vi "IMAQ Trigger the captured image.vi"() -> ()   [LabVIEW 2018]
uses:
  LabViewDVPCamera/LabViewDVPCamera.lvlib
panel:
  out "Image":T1(plugin-control)
  in  "Trigger":bool
  in  "CloseFlg":i32
  out "handle":u32
  in  "CameraList":u16(ring) items=["MGS130M-192.168.0.251"]
  in  "Set":bool
  in  "Close":bool
  in  "Open":bool
  in  "ScanCamera":bool
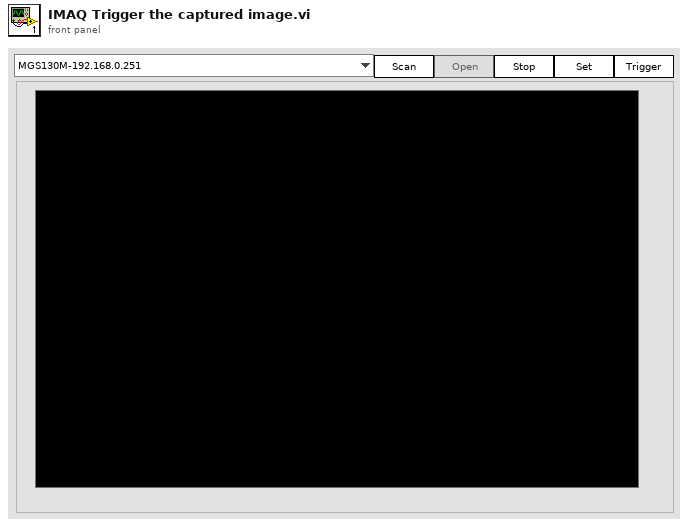
[diagram p1: front panel]
types:
  T1 = typedef "IMAQ Image.ctl" = refnum<image>
  T2 = enum8{"Enabled", "Disabled", "Disabled and Grayed Out"}
  T3 = typedef "LVStringsAndValuesArrayTypeDef_U16.ctl" = cluster{"String":string, "Value":u16}[]
  T4 = typedef "Image Type" = u32
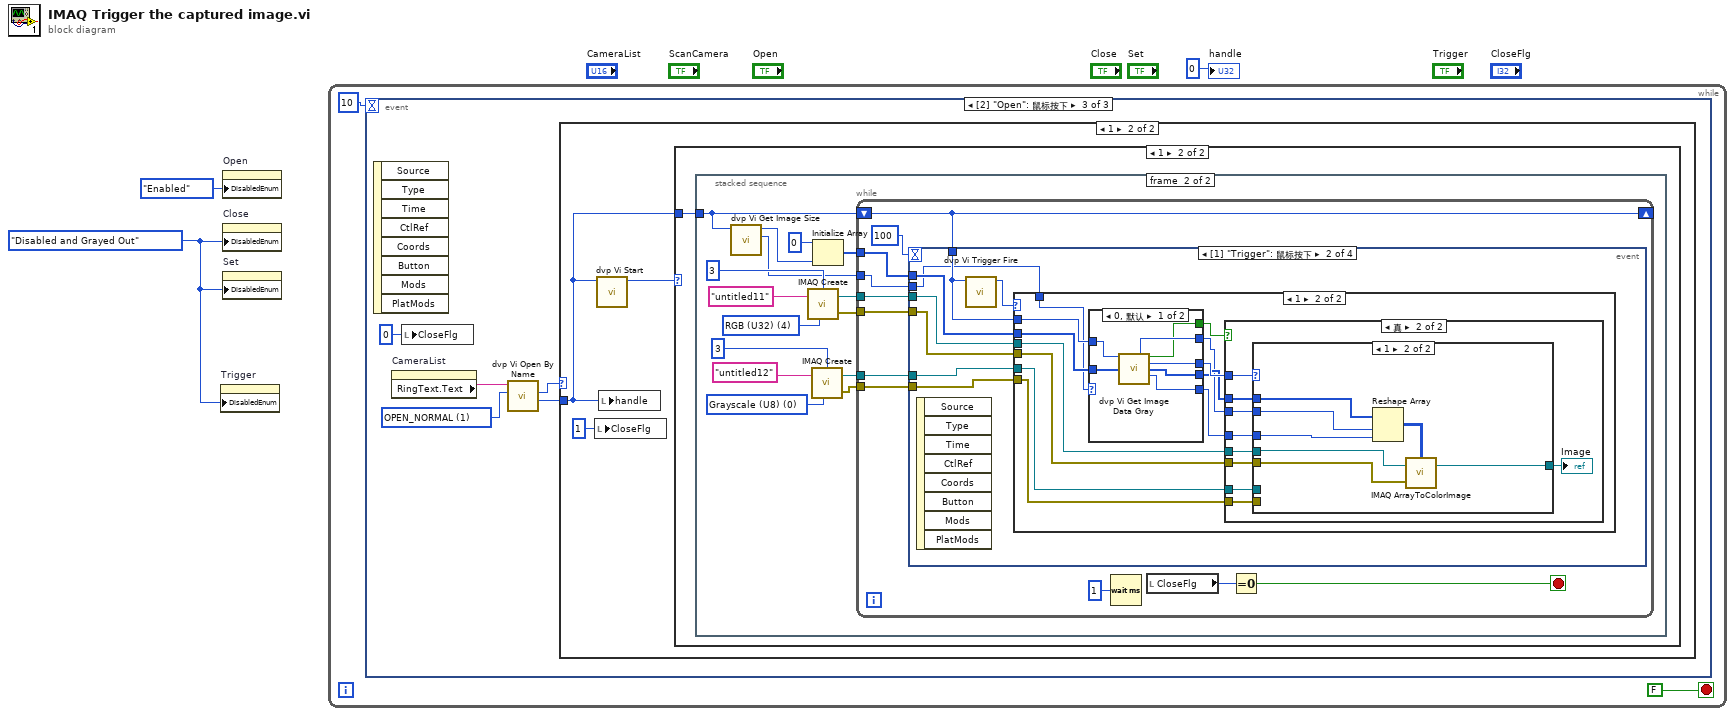
[diagram p0: block diagram]
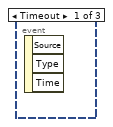
[diagram p2: hidden frame]
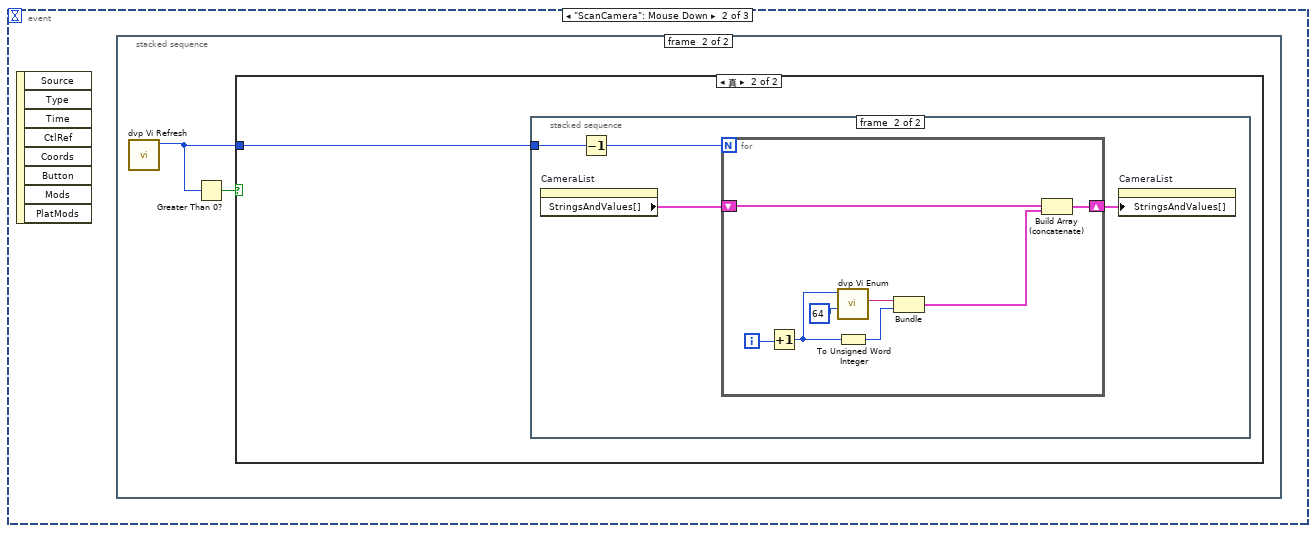
[diagram p3: hidden frame]
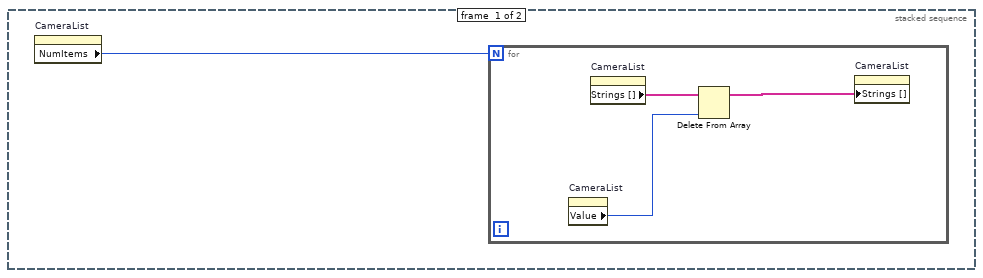
[diagram p4: hidden frame]
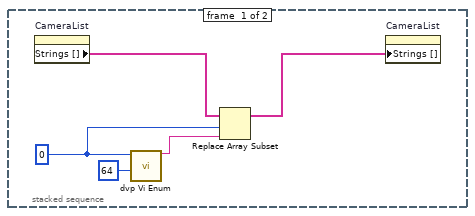
[diagram p6: hidden frame]
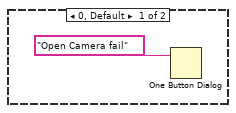
[diagram p7: hidden frame]
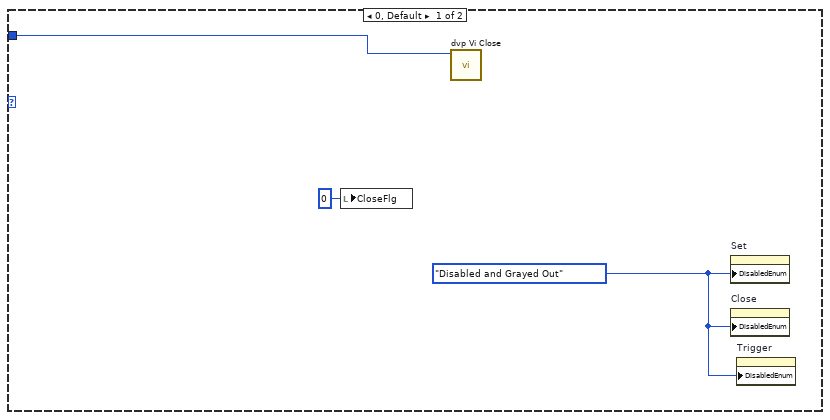
[diagram p8: hidden frame]
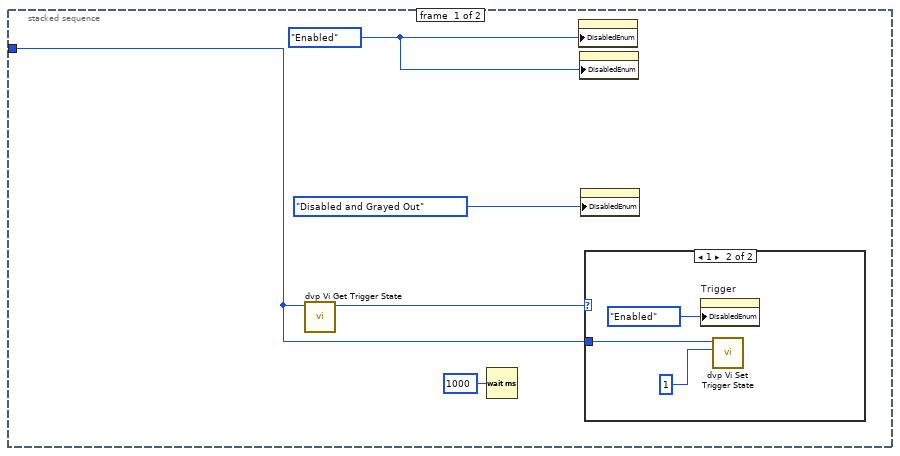
[diagram p9: hidden frame]
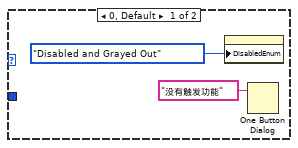
[diagram p10: hidden frame]
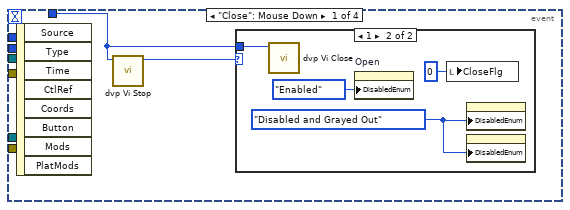
[diagram p11: hidden frame]
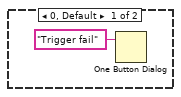
[diagram p13: hidden frame]
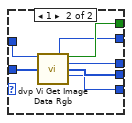
[diagram p14: hidden frame]
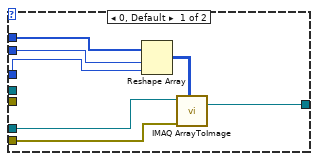
[diagram p16: hidden frame]
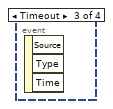
[diagram p17: hidden frame]
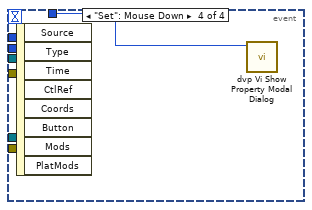
[diagram p18: hidden frame]
diagram:
  w1 = T2."Disabled and Grayed Out" ("禁用")
  n1 = property on="Trigger" class="Bool"("DisabledEnum"=w1) -> ()  [unwired: 2 in, 2 out]
  n2 = property on="Open" class="Bool"("DisabledEnum"=T2."Enabled" ("禁用")) -> ()  [unwired: 2 in, 2 out]
  n3 = property on="Close" class="Bool"("DisabledEnum"=w1) -> ()  [unwired: 2 in, 2 out]
  n4 = property on="Set" class="Bool"("DisabledEnum"=w1) -> ()  [unwired: 2 in, 2 out]
  n5 = while {
    stop <- FALSE stop-if-true
    n6 = event shown="[2] \"Open\": 鼠标按下" {
      selector: _ -> [_ _ _]
      dyn-events: _ -> [_ _ _]
      timeout: 10 -> [_ _ _]
      event Timeout {
        n7 = event-data() -> ()  [unwired: 1 in, 3 out]
      }
      event "ScanCamera": Mouse Down {
        n8 = event-data() -> ()  [unwired: 1 in, 8 out]
        n9 = stacked-sequence "清除下拉列表的数据" {
          frame #0 {
            n10 = property on="CameraList" class="Ring (严格)"() -> ("NumItems"=w6:u32)  [unwired: 2 in, 2 out]
            n11 = for {
              N: w6 -> [_]
              n12 = property on="CameraList" class="Ring (严格)"() -> ("Value"=w8:u16)  [unwired: 2 in, 2 out]
              n13 = property on="CameraList" class="Ring (严格)"() -> ("Strings []"=w7:string[])  [unwired: 2 in, 2 out]
              n14 = Delete From Array ("删除数组元素")(array=w7, index=w8) -> (array with subset deleted=w9:string[])  [unwired: 1 in, 1 out]
              n15 = property on="CameraList" class="Ring (严格)"("Strings []"=w9) -> ()  [unwired: 2 in, 2 out]
            }
          }
          frame #1 {
            n16 = call "dvp Vi Refresh.vi"() -> ("pCount out"=w11:u32)  [unwired: 10 in, 1 out]
            n17 = Greater Than 0?(x=w11) -> (x > 0?=w10:bool)
            n18 = case shown="真" w10 {
              tunnel: w11 -> [_ w12]
              frame False {
              }
              frame True {
                n19 = stacked-sequence {
                  tunnel: w12 -> [_ w19]
                  frame #0 {
                    w13 = u32 0 ("index")
                    n20 = property on="CameraList" class="Ring (严格)"() -> ("Strings []"=w16:string[])  [unwired: 2 in, 2 out]
                    n21 = call "dvp Vi Enum.vi"("unSize"=u32 64, "index"=w13) -> ("friendlyName out"=w15:string)  [unwired: 8 in, 1 out]
                    n22 = Replace Array Subset ("替换数组子集")(array=w16, new element=w15, index=w13) -> (w17:string[])
                    n23 = property on="CameraList" class="Ring (严格)"("Strings []"=w17) -> ()  [unwired: 2 in, 2 out]
                  }
                  frame #1 {
                    n24 = property on="CameraList" class="Ring (严格)"() -> ("StringsAndValues[]"=w21:T3)  [unwired: 2 in, 2 out]
                    n25 = Decrement(x=w19) -> (x-1=w18:u32)
                    n26 = for {
                      N: w18 -> [_]
                      shift-right: [w28] -> w20
                      shift-left: w21 -> [w26]
                      i -> [w23]
                      n27 = Increment(x=w23) -> (x+1=w22:i32)
                      n28 = call "dvp Vi Enum.vi"("unSize"=u32 64, "index"=w22) -> ("friendlyName out"=w29:string)  [unwired: 8 in, 1 out]
                      n29 = To Unsigned Word Integer(number=w22) -> (unsigned 16bit integer=w25:u16)
                      n30 = Bundle("friendlyName out"=w29, w25) -> (w27:cluster{"friendlyName out":string, u16})  [unwired: 1 in]
                      n31 = Build Array (concatenate)(w26, w27) -> (w28:T3)
                    }
                    n32 = property on="CameraList" class="Ring (严格)"("StringsAndValues[]"=w20) -> ()  [unwired: 2 in, 2 out]
                  }
                }
              }
            }
          }
        }
      }
      event "Open": Mouse Down {
        w32 = u32 1 items=["OPEN_OFFLINE", "OPEN_NORMAL"] ("type")
        n33 = event-data() -> ()  [unwired: 1 in, 8 out]
        n34 = property on="CameraList" class="Ring (严格)"() -> ("RingText.Text"=w31:string)  [unwired: 2 in, 2 out]
        n35 = local write "CloseFlg"(0 ("CloseFlg")) -> ()
        n36 = call "dvp Vi Open By Name.vi"("type"=w32, "friendlyName"=w31) -> ("pHandle out"=w34:u32, "function return"=w33:u32)  [unwired: 7 in, 1 out]
        n37 = case shown="1" w33 {
          tunnel: w34 -> [_ w38]
          frame 0, Default {
            n38 = One Button Dialog(message="Open Camera fail" ("消息")) -> ()  [unwired: 1 in, 1 out]
          }
          frame 1 {
            n39 = local write "CloseFlg"(1 ("CloseFlg")) -> ()
            n40 = call "dvp Vi Start.vi"("handle"=w38) -> ("function return"=w36:u32)  [unwired: 10 in]
            n41 = local write "handle"(w38) -> ()
            n42 = case shown="1" w36 {
              tunnel: w38 -> [w41 w42]
              frame 0, Default {
                w39 = T2."Disabled and Grayed Out" ("禁用")
                n43 = local write "CloseFlg"(0 ("CloseFlg")) -> ()
                n44 = call "dvp Vi Close.vi"("handle"=w41) -> ()  [unwired: 10 in, 1 out]
                n45 = property on="Set" class="Bool"("DisabledEnum"=w39) -> ()  [unwired: 2 in, 2 out]
                n46 = property on="Close" class="Bool"("DisabledEnum"=w39) -> ()  [unwired: 2 in, 2 out]
                n47 = property on="Trigger" class="Bool"("DisabledEnum"=w39) -> ()  [unwired: 2 in, 2 out]
              }
              frame 1 {
                n48 = stacked-sequence {
                  tunnel: w42 -> [w44 w55]
                  frame #0 {
                    w46 = T2."Enabled" ("禁用")
                    n49 = call "dvp Vi Get Trigger State.vi"("handle"=w44) -> ("function return"=w45:u32)  [unwired: 9 in, 1 out]
                    n50 = Wait (ms)(milliseconds to wait=u32 1000 ("等待时间（毫秒）")) -> ()  [unwired: 1 out]
                    n51 = property on="Set" class="Bool"("DisabledEnum"=w46) -> ()  [unwired: 2 in, 2 out]
                    n52 = property on="Close" class="Bool"("DisabledEnum"=w46) -> ()  [unwired: 2 in, 2 out]
                    n53 = property on="Open" class="Bool"("DisabledEnum"=T2."Disabled and Grayed Out" ("禁用")) -> ()  [unwired: 2 in, 2 out]
                    n54 = case shown="1" w45 {
                      tunnel: w44 -> [_ w51]
                      frame 0, Default {
                        n55 = property on="Trigger" class="Bool"("DisabledEnum"=T2."Disabled and Grayed Out" ("禁用")) -> ()  [unwired: 2 in, 2 out]
                        n56 = One Button Dialog(message="没有触发功能" ("消息")) -> ()  [unwired: 1 in, 1 out]
                      }
                      frame 1 {
                        n57 = property on="Trigger" class="Bool"("DisabledEnum"=T2."Enabled" ("禁用")) -> ()  [unwired: 2 in, 2 out]
                        n58 = call "dvp Vi Set Trigger State.vi"("TriggerState"=1, "handle"=w51) -> ()  [unwired: 9 in, 1 out]
                      }
                    }
                  }
                  frame #1 {
                    w61 = T4 0 items=["Grayscale (U8)", "Grayscale (I16)", "Grayscale (SGL)", "Complex (CSG)", "RGB (U32)", "HSL (U32)", "RGB (U64)", "Grayscale (U16)"] ("Image Type")
                    w65 = T4 4 items=["Grayscale (U8)", "Grayscale (I16)", "Grayscale (SGL)", "Complex (CSG)", "RGB (U32)", "HSL (U32)", "RGB (U64)", "Grayscale (U16)"] ("Image Type")
                    n59 = call "dvp Vi Get Image Size.vi"("handle"=w55) -> ("pformat out"=w53:i32, "function return"=w66:u32)  [unwired: 9 in]
                    n60 = call "IMAQ Create"("Border Size"=3, "Image Name"="untitled11", "Image Type"=w65) -> ("New Image"=w57:T1, "error out"=w56:errorcluster)  [unwired: 2 in]
                    n61 = call "IMAQ Create"("Border Size"=3, "Image Name"="untitled12", "Image Type"=w61) -> ("New Image"=w54:T1, "error out"=w58:errorcluster)  [unwired: 2 in]
                    n62 = Initialize Array(u32 0 ("元素"), w66) -> (w59:u32[])
                    n63 = while {
                      shift-right: [w74] -> _
                      shift-left: w55 -> [w74]
                      tunnel: w59 -> [w73]
                      tunnel: w58 -> [w69]
                      tunnel: w57 -> [w72]
                      tunnel: w56 -> [w71]
                      tunnel: w54 -> [w70]
                      tunnel: w53 -> [w68]
                      stop <- w77 stop-if-true
                      n64 = event shown="[1] \"Trigger\": 鼠标按下" {
                        selector: _ -> [_ _ _ _]
                        dyn-events: _ -> [_ _ _ _]
                        timeout: 100 -> [_ _ _ _]
                        tunnel: w74 -> [w79 w91 _ w143]
                        tunnel: w73 -> [_ w90 _ _]
                        tunnel: w72 -> [_ w87 _ _]
                        tunnel: w71 -> [_ w86 _ _]
                        tunnel: w70 -> [_ w89 _ _]
                        tunnel: w69 -> [_ w88 _ _]
                        tunnel: w68 -> [_ w85 _ _]
                        event "Close": Mouse Down {
                          n65 = event-data() -> ()  [unwired: 1 in, 8 out]
                          n66 = call "dvp Vi Stop.vi"("handle"=w79) -> ("function return"=w80:u32)  [unwired: 10 in]
                          n67 = case shown="1" w80 {
                            tunnel: w79 -> [_ w82]
                            frame 0, Default {
                            }
                            frame 1 {
                              w81 = T2."Disabled and Grayed Out" ("禁用")
                              n68 = call "dvp Vi Close.vi"("handle"=w82) -> ()  [unwired: 10 in, 1 out]
                              n69 = property on="Open" class="Bool"("DisabledEnum"=T2."Enabled" ("禁用")) -> ()  [unwired: 2 in, 2 out]
                              n70 = local write "CloseFlg"(0 ("CloseFlg")) -> ()
                              n71 = property on="Close" class="Bool"("DisabledEnum"=w81) -> ()  [unwired: 2 in, 2 out]
                              n72 = property on="Set" class="Bool"("DisabledEnum"=w81) -> ()  [unwired: 2 in, 2 out]
                            }
                          }
                        }
                        event "Trigger": Mouse Down {
                          n73 = event-data() -> ()  [unwired: 1 in, 8 out]
                          n74 = call "dvp Vi Trigger Fire.vi"("handle"=w91) -> ("function return"=w92:u32)  [unwired: 10 in]
                          n75 = case shown="1" w92 {
                            tunnel: w91 -> [_ w101]
                            tunnel: w90 -> [_ w100]
                            tunnel: w89 -> [_ w103]
                            tunnel: w88 -> [_ w102]
                            tunnel: w87 -> [_ w105]
                            tunnel: w86 -> [_ w104]
                            tunnel: w85 -> [_ w99]
                            frame 0, Default {
                              n76 = One Button Dialog(message="Trigger fail" ("消息")) -> ()  [unwired: 1 in, 1 out]
                            }
                            frame 1 {
                              n77 = case shown="0, 默认" w99 {
                                tunnel: w100 -> [w112 w119]
                                tunnel: w101 -> [w111 w118]
                                tunnel: [w107 w117] -> w98
                                tunnel: [w109 w116] -> w96
                                tunnel: [w108 w115] -> w97
                                tunnel: [w110 w114] -> w95
                                tunnel: [w106 w113] -> w94
                                frame 0, Default {
                                n78 = call "dvp Vi Get Image Data Gray.vi"("handle"=w111, "pbuffer"=w112) -> ("piHeight out"=w110:i32, "function return"=w107:bool, "pformat out"=w108:i32, "pbuffer out"=w109:u8[], "piWidth out"=w106:i32)  [unwired: 9 in]
                                }
                                frame 1 {
                                n79 = call "dvp Vi Get Image Data Rgb.vi"("handle"=w118, "pbuffer"=w119) -> ("piHeight out"=w114:i32, "function return"=w117:bool, "pformat out"=w115:i32, "pbuffer out"=w116:u32[], "piWidth out"=w113:i32)  [unwired: 9 in]
                                }
                              }
                              n80 = case shown="真" w98 {
                                tunnel: w94 -> [_ w128]
                                tunnel: w95 -> [_ w127]
                                tunnel: w96 -> [_ w126]
                                tunnel: w97 -> [_ w125]
                                tunnel: w105 -> [_ w121]
                                tunnel: w103 -> [_ w124]
                                tunnel: w102 -> [_ w123]
                                tunnel: w104 -> [_ w122]
                                frame False {
                                }
                                frame True {
                                n81 = case shown="1" w125 {
                                tunnel: w127 -> [w135 w141]
                                tunnel: w128 -> [w134 w142]
                                tunnel: [w133 w139] -> w120
                                tunnel: w126 -> [w129 w138]
                                tunnel: w124 -> [w130 _]
                                tunnel: w123 -> [w131 _]
                                tunnel: w122 -> [_ w136]
                                tunnel: w121 -> [_ w137]
                                frame 0, Default {
                                n82 = Reshape Array ("重排数组维数")(w129, w135, w134) -> (w132:u32[][])
                                n83 = call "IMAQ ArrayToImage"("error in (no error)"=w131, "Image Pixels (U8)"=w132, "Image"=w130) -> ("Image Out"=w133:T1)  [unwired: 7 in, 1 out]
                                }
                                frame 1 {
                                n84 = Reshape Array ("重排数组维数")(w138, w141, w142) -> (w140:u32[][])
                                n85 = call "IMAQ ArrayToColorImage"("Image Pixels (U32)"=w140, "Image"=w137, "error in (no error)"=w136) -> ("Image Out"=w139:T1)  [unwired: 2 in, 1 out]
                                }
                                }
                                "Image" <- w120
                                }
                              }
                            }
                          }
                        }
                        event Timeout {
                          n86 = event-data() -> ()  [unwired: 1 in, 3 out]
                        }
                        event "Set": Mouse Down {
                          n87 = event-data() -> ()  [unwired: 1 in, 8 out]
                          n88 = call "dvp Vi Show Property Modal Dialog.vi"("handle"=w143) -> ()  [unwired: 10 in, 1 out]
                        }
                      }
                      n89 = Wait (ms)(milliseconds to wait=u32 1 ("等待时间（毫秒）")) -> ()  [unwired: 1 out]
                      n90 = local read "CloseFlg"() -> (w76:i32)
                      n91 = Equal To 0?(x=w76) -> (x = 0?=w77:bool)
                    }
                  }
                }
              }
            }
          }
        }
      }
    }
  }
  "handle" <- u32 0 ("handle")
